vi "Analysis Results.vi"(6 "Image Nr.":i32, 8 "error in (no error)":errorcluster, 9 "Results In":refnum<class "Analyze Results Base.lvclass">[](array[class]), 10 "Parameters":refnum<class "Analyze Parameter Base.lvclass">[](array[class]), 11 "Launch IMAQ Display in":refnum<class "HIJ Vision Application.lvclass">) -> (0 "error out":errorcluster, 3 "Launch IMAQ Display out":refnum<class "HIJ Vision Application.lvclass">)   [LabVIEW 2020, in "HIJ Vision Application.lvlib" / "HIJ Vision Application.lvclass"]
uses:
  HIJ Vision Application.lvclass
  HIJ Vision Application.lvclass/HIJ Vision Application.ctl
  Analyze/Results and Overlays/Results Base/Analyze Results Base.lvclass
  Analyze/Analyze Actor/IAnalysis Messages/Analysis Results Msg/Analysis Results Msg.lvclass
  Analyze/Analyze Parameter/Analyze Parameter Base/Analyze Parameter Base.lvclass
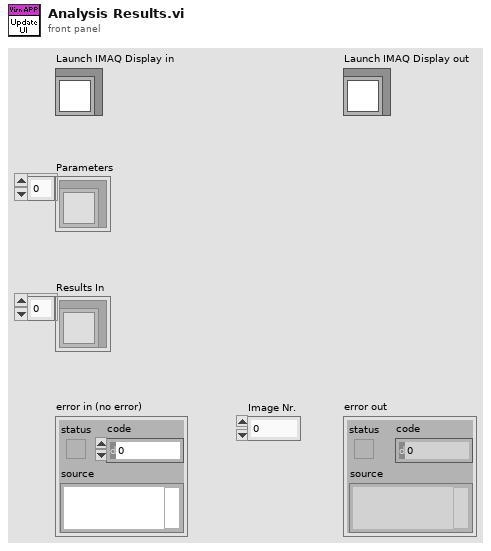
[diagram p1: front panel]
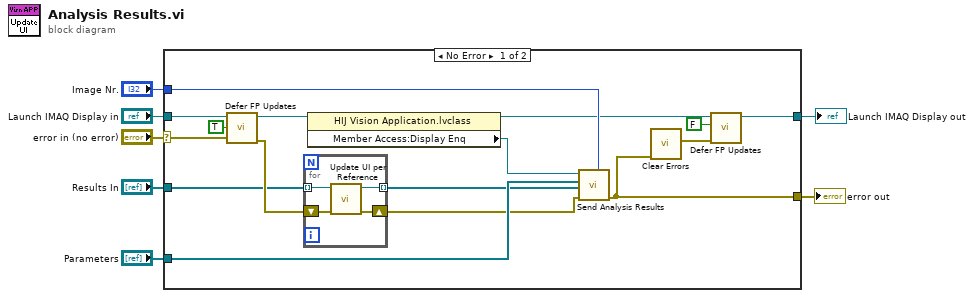
[diagram p0: block diagram]
diagram:
  n1 = case shown="No Error" "error in (no error)" {
    selector: "error in (no error)" -> [w20 w29]
    tunnel: [w9 w29] -> w6
    tunnel: [w16 w28] -> w4
    tunnel: "Launch IMAQ Display in" -> [w22 w28]
    tunnel: "Parameters" -> [w12 _]
    tunnel: "Results In" -> [w17 _]
    tunnel: "Image Nr." -> [w23 _]
    frame No Error {
      n2 = call-dynamic "Defer FP Updates.vi"("error in (no error)"=w20, "Disable"=TRUE, "ViewableActor in"=w22) -> ("error out"=w19:errorcluster, "ViewableActor out"=w21:refnum<class "HIJ Vision Application.lvclass">)  [unwired: 7 in]
      n3 = for {
        tunnel: w17 -> [w27] mode=indexing
        shift-right: [w25] -> w10
        shift-left: w19 -> [w26]
        tunnel: [w24] -> w11 mode=indexing
        n4 = call-dynamic "Update UI per Reference.vi"("error in (no error)"=w26, "Analyze Results Base in"=w27) -> ("error out"=w25:errorcluster, "Analyze Results Base out"=w24:refnum<class "Analyze Results Base.lvclass">)  [unwired: 8 in]
      }
      n5 = property class="HIJ Vision Application.lvclass"(reference=w21) -> (reference out=w14:refnum<class "HIJ Vision Application.lvclass">, "Member Access:Display Enq"=w13:refnum<class "Message Enqueuer.lvclass">)  [unwired: 1 in, 1 out]
      n6 = call "Send Analysis Results.vi"("Image Nr."=w23, "error in (no error)"=w10, "Results In"=w11, "Parameters"=w12, "Message Enqueuer"=w13) -> ("error out"=w9:errorcluster)  [unwired: 5 in, 1 out]
      n7 = call <vilib>:"Clear Errors.vi"("error in (no error)"=w9) -> ("error out"=w15:errorcluster)  [unwired: 5 in, 1 out]
      n8 = call-dynamic "Defer FP Updates.vi"("error in (no error)"=w15, "Disable"=FALSE, "ViewableActor in"=w14) -> ("ViewableActor out"=w16:refnum<class "HIJ Vision Application.lvclass">)  [unwired: 7 in, 1 out]
    }
    frame Error {
    }
  }
  "error out" <- w6
  "Launch IMAQ Display out" <- w4
